vi "Write Alarm Status.vi"(8 "error in":errorcluster, 10 "alarm status":T1, 11 "PV Data in":refnum<class "PV Data.lvclass">) -> (0 "error out":errorcluster, 3 "PV Data out":refnum<class "PV Data.lvclass">)   [LabVIEW 2020, in "PV Access.lvlib" / "PV Data.lvlib" / "PV Data.lvclass"]
uses:
  PV Data.lvclass
  PV Access.lvlib
  Alarm.ctl
  PV Data.lvlib
  Alarm Severity.ctl
  Alarm Status.ctl
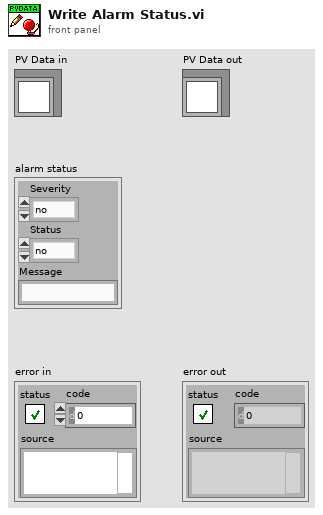
[diagram p1: front panel]
types:
  T1 = typedef "PV Access.lvlib/PV Data.lvlib/Alarm.ctl" = cluster{"Severity":T2, "Status":T3, "Message":string}
  T2 = typedef "PV Access.lvlib/PV Data.lvlib/Alarm Severity.ctl" = enum32{"no", "minor", "major", "record", "invalid", "undefined", ""}
  T3 = typedef "PV Access.lvlib/PV Data.lvlib/Alarm Status.ctl" = enum32{"no", "device", "driver", "record", "db", "conf", "undefined", "client"}
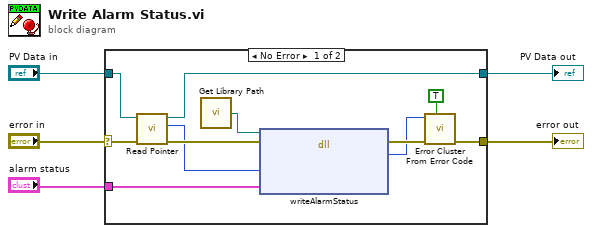
[diagram p0: block diagram]
diagram:
  n1 = case shown="No Error" "error in" {
    selector: "error in" -> [w11 w18]
    tunnel: [w12 w18] -> w5
    tunnel: "PV Data in" -> [w9 w17]
    tunnel: [w7 w17] -> w2
    tunnel: "alarm status" -> [w6 _]
    frame No Error {
      n2 = call-dynamic "Read Pointer.vi"("error in (no error)"=w11, "Pointer Base in"=w9) -> ("error out"=w10:errorcluster, "Pointer"=w8:i64, "Pointer Base out"=w7:refnum<class "PV Data.lvclass">)  [unwired: 7 in]
      n3 = call "Get Library Path.vi"() -> ("Path"=w16:path)  [unwired: 1 in]
      n4 = dll-call lib="?" fn="writeAlarmStatus"(path in=w16, error in=w10, "value"=w8, "alarm status"=w6) -> (error out=w14:errorcluster, "err_code"=w13:i32)  [unwired: 3 in, 1 out]
      n5 = call <vilib>:"Error Cluster From Error Code.vi"("show call chain? (False)"=TRUE, "error in (no error)"=w14, "error code (0)"=w13) -> ("error out"=w12:errorcluster)  [unwired: 6 in]
    }
    frame Error {
    }
  }
  "error out" <- w5
  "PV Data out" <- w2
